vi "Bezier Curve.vi"(1 "Step":i32=10, 2 "Data In":dbl[][](array[numeric])) -> (0 "Data Out":dbl[][](array[numeric]))   [LabVIEW 2017]
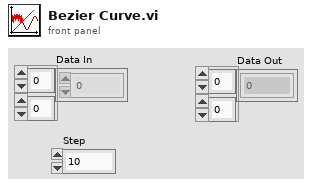
[diagram p1: front panel]
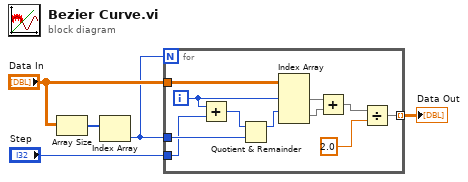
[diagram p0: block diagram]
diagram:
  n1 = Array Size(array="Data In") -> (size(s)=w5:i32[])
  n2 = Index Array(array=w5) -> (element=w3:i32)  [unwired: 1 in]
  n3 = for {
    N: w3 -> [_]
    tunnel: "Data In" -> [w14]
    tunnel: w3 -> [w15]
    tunnel: [w7] -> w2 mode=indexing
    tunnel: "Step" -> [w6]
    i -> [w13]
    n4 = Add(x=w13, y=w6) -> (x+y=w16:i32)
    n5 = Quotient & Remainder(x=w16, y=w15) -> (x-y*floor(x/y)=w12:i32)  [unwired: 1 out]
    n6 = Index Array(array=w14, index (row) #1=w13, index (row) #2=w12) -> (element #1=w11:dbl[], element #2=w10:dbl[])  [unwired: 2 in]
    n7 = Add(x=w11, y=w10) -> (x+y=w9:dbl[])
    n8 = Divide(x=w9, y=2.0) -> (x/y=w7:dbl[])
  }
  "Data Out" <- w2
